vi "Store Number  (SubVI).vi"(9 "Command":T1=enum."Initialize", 11 "Numeric":dbl) -> (3 "Array":dbl[](array[numeric]))   [LabVIEW 2019]
uses:
  control/command control.ctl
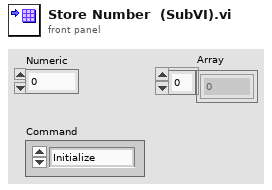
[diagram p1: front panel]
types:
  T1 = typedef "command control.ctl" = enum16{"Multiply", "Divide", "Initialize", "Minus", "Equal", "Add", "Decimal Point", "Number"}
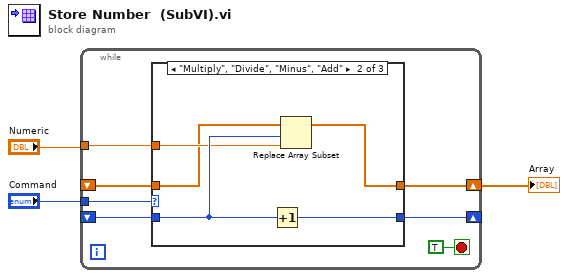
[diagram p0: block diagram]
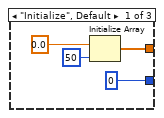
[diagram p2: hidden frame]
diagram:
  n1 = while {
    shift-right: [w9] -> w2
    shift-left: _ -> [w8]
    tunnel: "Command" -> [w7]
    shift-right: [w6] -> _
    shift-left: _ -> [w5]
    tunnel: "Numeric" -> [w4]
    stop <- TRUE stop-if-true
    n2 = case shown="\"Multiply\", \"Divide\", \"Minus\", \"Add\"" w7 {
      tunnel: [w14 w15 w21] -> w9
      tunnel: w8 -> [_ w16 w21]
      tunnel: [0 ("dimension size") w19 w20] -> w6
      tunnel: w5 -> [_ w18 w20]
      tunnel: w4 -> [_ w17 _]
      frame "Initialize", Default {
        n3 = Initialize Array(0.0, 50 ("dimension size")) -> (w14:dbl[])
      }
      frame "Multiply", "Divide", "Minus", "Add" {
        n4 = Increment(x=w18) -> (x+1=w19:i32)
        n5 = Replace Array Subset(array=w16, new element=w17, index=w18) -> (w15:dbl[])
      }
      frame "Equal" {
      }
    }
  }
  "Array" <- w2
